vi "TDS Base Get Reference.vi"(8 "error in (no error)":errorcluster, 11 "Address":string) -> (0 "error out":errorcluster, 3 "Reference":refnum<visa-resource-name>)   [LabVIEW 2025, in "Interface Functions.lvlib"]
uses:
  Interface Functions.lvlib
panel:
  # "Get Reference"
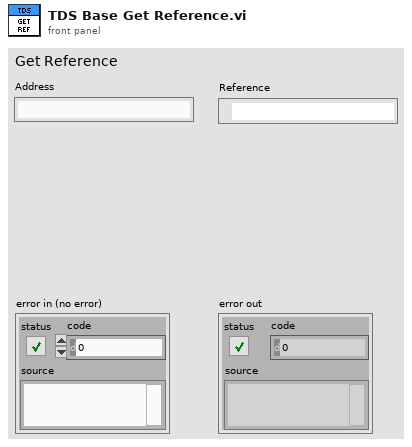
[diagram p1: front panel]
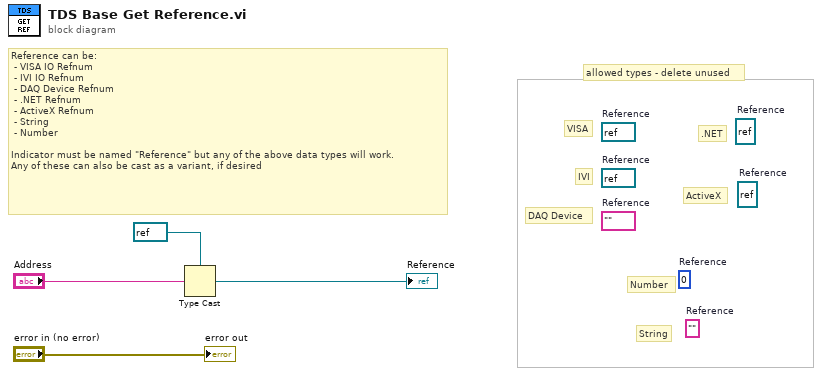
[diagram p0: block diagram]
diagram:
  (unwired) refnum<k7> refnum  # Reference
  (unwired) refnum<k24> refnum  # Reference
  (unwired) ""  # Reference
  (unwired) u64 0  # Reference
  (unwired) tag ""  # Reference
  (unwired) refnum<k15> refnum  # Reference
  (unwired) refnum<visa-resource-name> refnum  # Reference
  # "allowed types - delete unused"
  # "ActiveX"
  # "String"
  # "Number"
  # ".NET"
  # "DAQ Device"
  # "IVI"
  # "VISA"
  # "Reference can be:\n - VISA IO Refnum\n - IVI IO Refnum\n - DAQ Device Refnum\n - .NET Refnum\n - ActiveX Refnum\n - String\n - Number\n\nIndicator must be named \"Reference\" but any of the above data types will work.\nAny of these can also be cast as a variant, if desired"
  n1 = Type Cast(type=refnum<visa-resource-name> refnum ("Reference"), x="Address") -> (*(type *) &x=→"Reference":refnum<visa-resource-name>)
  "error out" <- "error in (no error)"
